vi "1. Basic Demo.vi"() -> ()   [LabVIEW 2020, in "1. Basic Panels.lvlib"]
doc: "This is the top level VI for this example. It will launch a variety of other panels.\n----\nCopyright: MGI 2017\nAuthor: Derek Trepanier"
uses:
  1. Basic Panels.lvlib
  <vilib>/MGI/Panel Manager/Panel/Panel/Window/Window.lvclass
  C:/Program Files/National Instruments/LabVIEW 2020/vi.lib/MGI/Panel Manager/Panel/Panel/Panel.lvclass
  <vilib>/MGI/Panel Manager/Panel/Panel/Window/Dialog/Dialog.lvclass
  <vilib>/MGI/Panel Manager/Panel/Panel/Subpanel/Subpanel.lvclass
  <vilib>/MGI/Panel Manager/Panel/Panel/Window/Window.vi
  <vilib>/MGI/Panel Manager/Panel/Panel/Window/Dialog/Dialog.vi
  <vilib>/MGI/Panel Manager/Panel/Panel/Subpanel/Subpanel.vi
  <vilib>/MGI/Panel Manager/Panel/Panel.lvlib
  <vilib>/MGI/Panel Manager/Panel/Panel/Panel.lvclass
panel:
  in  "Show Window":bool
  in  "Show Dialog":bool
  in  "Running Sub-Panels":i32(listbox)
  in  "New Subpanel Item":bool
  # "Windows"
  # "Run this VI to view a Panel Manager demo."
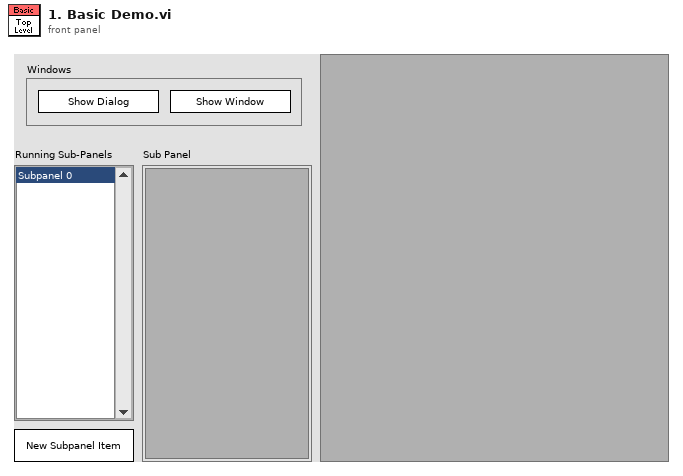
[diagram p1: front panel]
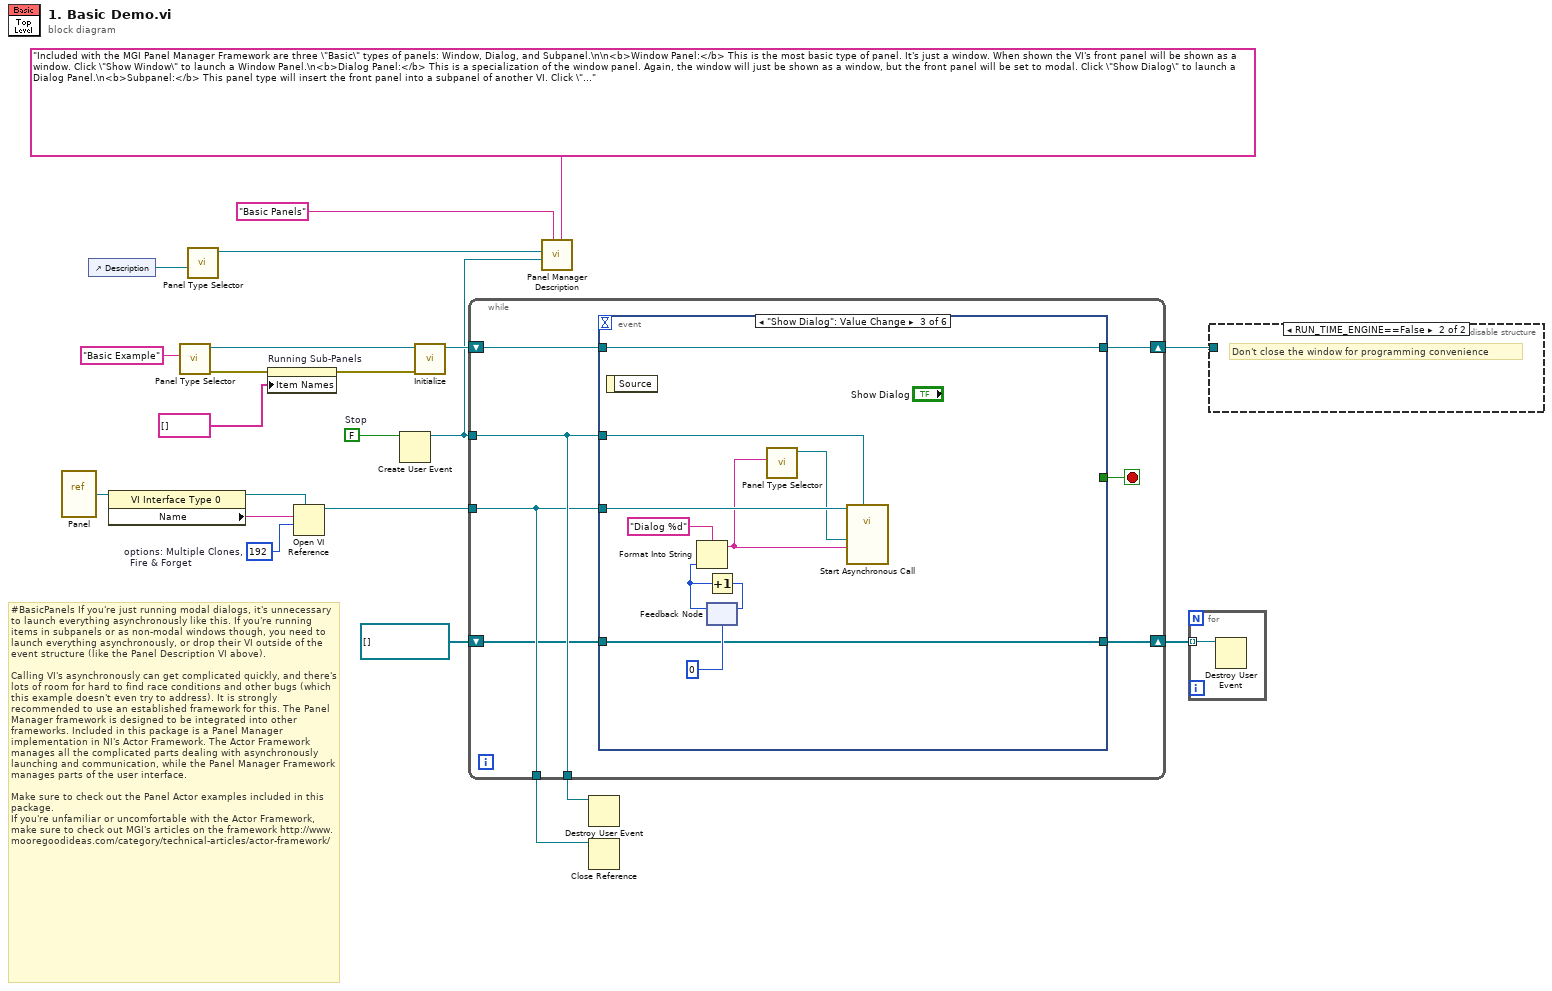
[diagram p0: block diagram]
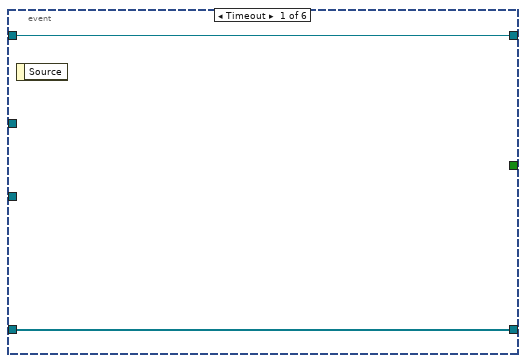
[diagram p2: hidden frame]
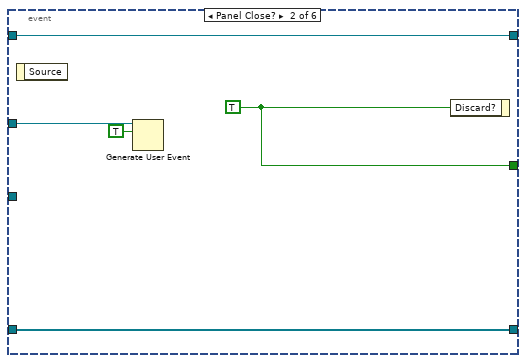
[diagram p3: hidden frame]
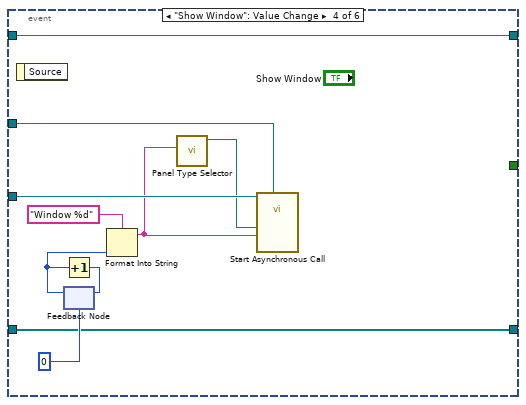
[diagram p4: hidden frame]
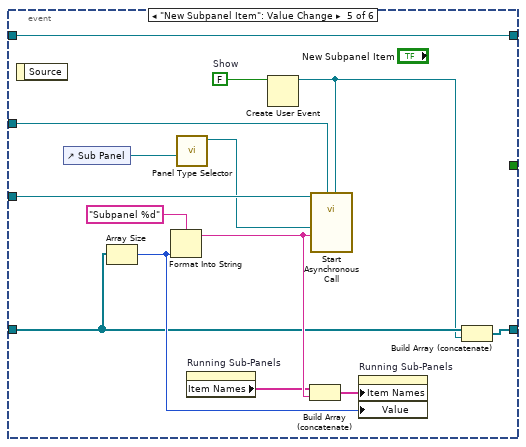
[diagram p5: hidden frame]
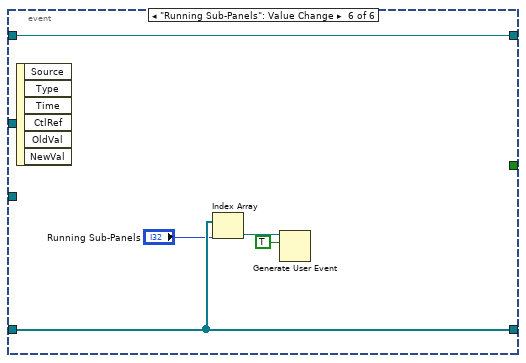
[diagram p6: hidden frame]
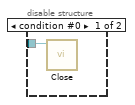
[diagram p7: hidden frame]
diagram:
  w12 = 192  # options: Multiple Clones,   Fire & Forget
  w19 = FALSE  # Stop
  # "#BasicPanels If you're just running modal dialogs, it's unnecessary to launch everything asynchronously like this. If you're running items in subpanels or as non-modal windows though, you need to launch everything asynchronously, or drop their VI outside of the event structure (like the Panel Description VI above).\n\nCalling VI's asynchronously can get complicated quickly, and there's lots of room for hard to find race conditions and other bugs (which this example doesn't even try to address). It is strongly recommended to use an established framework for this. The Panel Manager framework is designed to be integrated into other frameworks. Included in this package is a Panel Manager implementation in NI's Actor Framework. The Actor Framework manages all the complicated parts dealing with asynchronously launching and communication, while the Panel Manager Framework manages parts of the user interface.\n\nMake sure to check out the Panel Actor examples included in this package.\nIf you're unfamiliar or uncomfortable with the Actor Framework, make sure to check out MGI's articles on the framework http://www.mooregoodideas.com/category/technical-articles/actor-framework/"
  n1 = vi-ref "Panel.vi"() -> (w16:refnum<vi>)
  n2 = control-ref of="Description"() -> (w4:refnum<vi>)
  n3 = property class="VI Interface Type 0"(reference=w16) -> (reference out=w15:refnum<vi>, "Name"=w14:string)  [unwired: 1 in, 1 out]
  n4 = call-poly <vilib>:"Panel Type Selector.vi"("Default Title"="Basic Example" ("Title")) -> ("error out"=w10:errorcluster, "Window out"=w21:refnum<class "Window.lvclass">)  [unwired: 9 in]
  n5 = call-poly <vilib>:"Panel Type Selector.vi"("Sub Panel"=w4) -> ("Subpanel Out"=w5:refnum<class "Subpanel.lvclass">)  [unwired: 9 in, 1 out]
  n6 = property on="Running Sub-Panels" class="LstBox (strict)"(error in=w10, "Item Names"=string[] []) -> (error out=w9:errorcluster)  [unwired: 1 in, 1 out]
  n7 = Open VI Reference(type specifier VI Refnum (for type only)=w15, vi path=w14, options=w12) -> (vi reference=w13:refnum<vi>)  [unwired: 3 in, 1 out]
  n8 = Create User Event(user event datatype=w19) -> (user event=w3:refnum<user-event>)  [unwired: 1 in, 1 out]
  n9 = call <vilib>:"Initialize.vi"("error in (no error)"=w9, "Panel In"=w21) -> ("Panel Out"=w20:refnum<class "Window.lvclass">)  [unwired: 7 in, 2 out]
  n10 = while {
    shift-right: [w29] -> w18
    shift-left: w20 -> [w28]
    tunnel: w3 -> [w26]
    tunnel: [w26] -> w17
    tunnel: w13 -> [w25]
    tunnel: [w25] -> w11
    shift-right: [w24] -> w6
    shift-left: refnum<user-event>[] [] -> [w23]
    stop <- w27 stop-if-true
    n11 = event shown="[2] \"Show Dialog\": Value Change" {
      selector: _ -> [_ _ _ _ _ _]
      dyn-events: _ -> [_ _ _ _ _ _]
      timeout: _ -> [_ _ _ _ _ _]
      tunnel: [w31 w34 w39 w49 w66 w75] -> w29
      tunnel: w28 -> [w31 w34 w39 w49 w66 w75]
      tunnel: w26 -> [_ w36 w45 w55 w69 _]
      tunnel: [_ w33 _ _ _ _] -> w27
      tunnel: w25 -> [_ _ w46 w56 w70 _]
      tunnel: [w30 w32 w37 w47 w59 w74] -> w24
      tunnel: w23 -> [w30 w32 w37 w47 w60 w74]
      event Timeout {
        n12 = event-data() -> ()  [unwired: 1 in, 1 out]
      }
      event Panel Close? {
        w33 = TRUE ("Discard?")
        n13 = event-data() -> ()  [unwired: 1 in, 1 out]
        n14 = Generate User Event(user event=w36, event data cluster=TRUE ("event data")) -> ()  [unwired: 2 in, 2 out]
        n15 = event-data("Discard?"=w33) -> ()  [unwired: 1 in, 1 out]
      }
      event "Show Dialog": Value Change {
        n16 = event-data() -> ()  [unwired: 1 in, 1 out]
        n17 = feedback #1(0) -> (w42:i32)
        n18 = Format Into String(format string="Dialog %d", w42) -> (resulting string=w40:string)  [unwired: 2 in, 1 out]
        n19 = Increment(x=w42) -> (x+1=w43:i32)
        n20 = feedback-in #1(w43) -> ()
        n21 = call-poly <vilib>:"Panel Type Selector.vi"("Default Title"=w40) -> ("Dialog out"=w38:refnum<class "Dialog.lvclass">)  [unwired: 9 in, 1 out]
        n22 = call-by-ref "Start Asynchronous Call"(reference=w46, "Stop Event"=w45, "Label"=w40, "Panel"=w38) -> ()  [unwired: 10 in, 2 out]
      }
      event "Show Window": Value Change {
        n23 = event-data() -> ()  [unwired: 1 in, 1 out]
        n24 = feedback #2(0) -> (w52:i32)
        n25 = Increment(x=w52) -> (x+1=w53:i32)
        n26 = feedback-in #2(w53) -> ()
        n27 = Format Into String(format string="Window %d", w52) -> (resulting string=w50:string)  [unwired: 2 in, 1 out]
        n28 = call-poly <vilib>:"Panel Type Selector.vi"("Default Title"=w50) -> ("Window out"=w48:refnum<class "Window.lvclass">)  [unwired: 9 in, 1 out]
        n29 = call-by-ref "Start Asynchronous Call"(reference=w56, "Stop Event"=w55, "Label"=w50, "Panel"=w48) -> ()  [unwired: 10 in, 2 out]
      }
      event "New Subpanel Item": Value Change {
        w64 = FALSE  # Show
        n30 = event-data() -> ()  [unwired: 1 in, 1 out]
        n31 = control-ref of="Sub Panel"() -> (w65:refnum<vi>)
        n32 = Array Size(array=w60) -> (size(s)=w61:i32)
        n33 = Format Into String(format string="Subpanel %d", w61) -> (resulting string=w63:string)  [unwired: 2 in, 1 out]
        n34 = call-poly <vilib>:"Panel Type Selector.vi"("Sub Panel"=w65) -> ("Subpanel Out"=w67:refnum<class "Subpanel.lvclass">)  [unwired: 9 in, 1 out]
        n35 = property on="Running Sub-Panels" class="LstBox (strict)"() -> ("Item Names"=w57:string[])  [unwired: 2 in, 2 out]
        n36 = Create User Event(user event datatype=w64) -> (user event=w58:refnum<user-event>)  [unwired: 1 in, 1 out]
        n37 = Build Array (concatenate)(w57, w63) -> (w62:string[])
        n38 = call-by-ref "Start Asynchronous Call"(reference=w70, "Show Event"=w58, "Stop Event"=w69, "Label"=w63, "Panel"=w67) -> ()  [unwired: 9 in, 2 out]
        n39 = property on="Running Sub-Panels" class="LstBox (strict)"("Item Names"=w62, "Value"=w61) -> ()  [unwired: 2 in, 2 out]
        n40 = Build Array (concatenate)(w60, w58) -> (w59:refnum<user-event>[])
      }
      event "Running Sub-Panels": Value Change {
        n41 = event-data() -> ()  [unwired: 1 in, 6 out]
        n42 = Index Array(array=w74, index="Running Sub-Panels") -> (element=w72:refnum<user-event>)
        n43 = Generate User Event(user event=w72, event data cluster=TRUE ("event data")) -> ()  [unwired: 2 in, 2 out]
      }
    }
  }
  n44 = call "Panel Manager Description.vi"("Description"="Included with the MGI Panel Manager Framework are three \"Basic\" types of panels: Window, Dialog, and Subpanel.\n\n<b>Window Panel:</b> This is the most basic type of panel. It's just a window. When shown the VI's front panel will be shown as a window. Click \"Show Window\" to launch a Window Panel.\n<b>Dialog Panel:</b> This is a specialization of the window panel. Again, the window will just be shown as a window, but the front panel will be set to modal. Click \"Show Dialog\" to launch a Dialog Panel.\n<b>Subpanel:</b> This panel type will insert the front panel into a subpanel of another VI. Click \"New Subpanel Item\" to launch a new Subpanel Panel. The list of running subpanel items is show in the \"Running Sub-Panels\" Listbox.\n\nView the #BasicPanels bookmark for more info.", "Description Title"="Basic Panels", "Stop Event"=w3, "Panel"=w5) -> ()  [unwired: 7 in, 1 out]
  n45 = Destroy User Event(user event=w17) -> ()  [unwired: 1 in, 1 out]
  n46 = Close Reference(reference=w11) -> ()  [unwired: 1 in, 1 out]
  n47 = for {
    tunnel: w6 -> [w76] mode=indexing
    n48 = Destroy User Event(user event=w76) -> ()  [unwired: 1 in, 1 out]
  }
  n49 = disable-structure shown="RUN_TIME_ENGINE==False" {
    disable-tunnel: w18 -> [w77 _]
    frame condition #0 {
      n50 = call-dynamic "Close.vi"("UI Element in"=w77) -> ()  [unwired: 10 in, 1 out]
    }
    frame condition #1 (active) {
      # "Don't close the window for programming convenience"
    }
  }
